vi "Configuration.vi"() -> ()   [LabVIEW 2018]
panel:
  in  "Density [kg/m] 4":dbl
  in  "Fuel Type 4":T1(ring)
  in  "Diameter [m] 4":dbl
  in  "Height [m] 4":dbl
  in  "Density [kg/m] 3":dbl
  in  "Fuel Type 3":T1(ring)
  in  "Diameter [m] 3":dbl
  in  "Height [m] 3":dbl
  in  "Density [kg/m] 2":dbl
  in  "Fuel Type 2":T1(ring)
  in  "Diameter [m] 2":dbl
  in  "Height [m] 2":dbl
  in  "Density [kg/m]":dbl
  in  "Fuel Type":T1(ring)
  in  "Diameter [m]":dbl
  in  "Height [m]":dbl
  in  "stop":bool
  # "Tank 4 Parameters"
  # "Tank 3 Parameters"
  # "Tank 2 Parameters"
  # "Tank 1 Parameters"
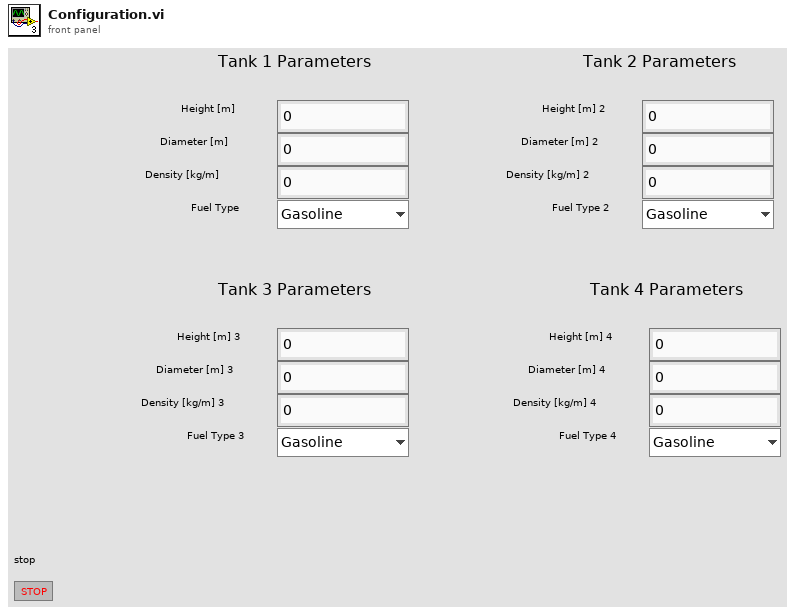
[diagram p1: front panel]
types:
  T1 = enum16{"Gasoline", "Diesel", "Kerosene", "Crude Oil"}
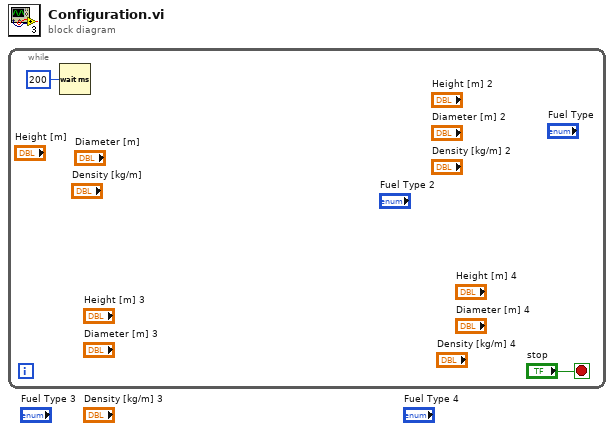
[diagram p0: block diagram]
diagram:
  n1 = while {
    stop <- "stop" stop-if-true
    n2 = Wait (ms)(milliseconds to wait=u32 200) -> ()  [unwired: 1 out]
  }
